vi "CalibrateMultiFlows.vi"(6 "Base Dilution":dbl=0.1, 7 "MFCS_EZ":T4=refnum, 8 "Manual Default Set Pressures":dbl[](array[numeric])=[268.25189208984375, 1037.0302734375, 980.2239990234375, 978.9616088867188], 9 "Missaleneouns Parems":T2={"Ctr Odor Valve"=14, "Water Mix Valve"=12, "Total Odor Flow"=425.0, "Total Flow Setpoint"=531.25, "Control Pressure Channel"=1, "Mix Water Pressure Channel"=2}, 10 "Calibration Refs":T3={"Pressure Controller List"=[2, 2, 2, 3, 4], "Ratio List"=[0.9, 0.7, 0.6, 0.1, 0.1], "Valve List"=[12, 12, 12, 0, 8]}, 11 "Calibration Mode":T5(ring)) -> (0 "Aborted?":bool, 2 "New Manual Pressure":dbl[](array[numeric]), 3 "Set Pressure Cluster":T1)   [LabVIEW 2016]
uses:
  <userlib>/Fluigent/Fluigent MFCS/FluigentMFCS_Full.llb/_EZmfcsRefNum.ctl
  <userlib>/Fluigent/Fluigent MFCS/FluigentMFCS_Full.llb/_EZmfcsEnum.ctl
  <userlib>/Fluigent/Fluigent MFCS/FluigentMFCS_Full.llb/MFCS_EZ Write Channel Pressure.vi
panel:
  out "Set Water Mix Pressures":dbl[](array[numeric])
  out "Control Pressure":dbl=268.25189208984375
  out "odor Starting Pressure":dbl=980.2239990234375
  out "Water Mix Starting PRessure":dbl=1037.0302734375
  out "Ctr Starting Pressure":dbl=268.25189208984375
  out "Set Odor Pressures":dbl[](array[numeric])
  # "Indexed by pressure controller"
  # "indexed by possible ratios"
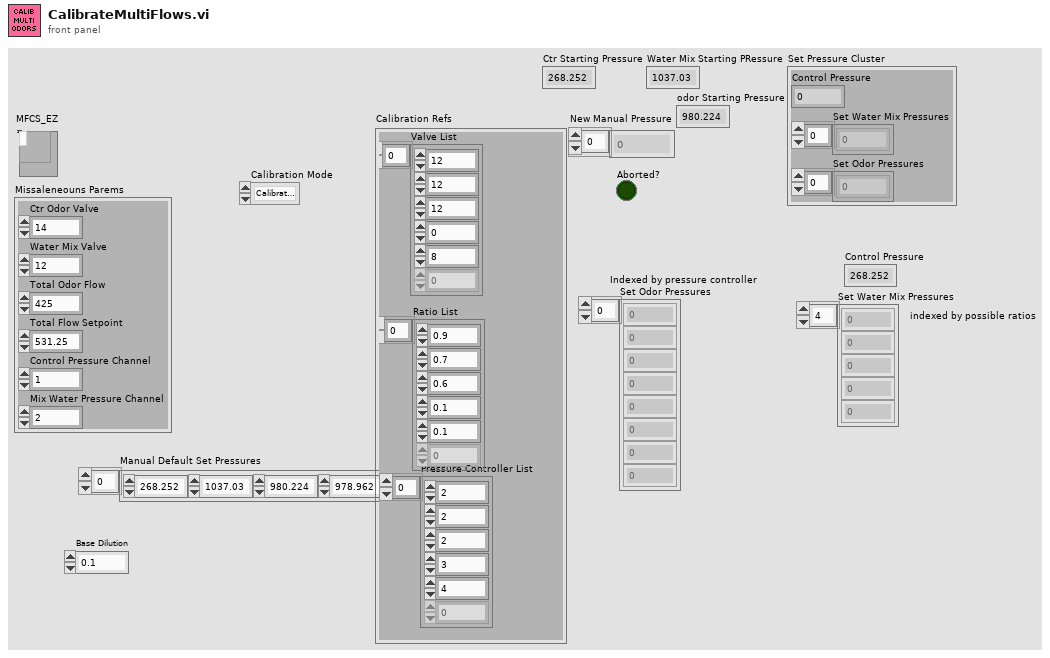
[diagram p1: front panel]
types:
  T1 = cluster{"Control Pressure":dbl, "Set Water Mix Pressures":dbl[], "Set Odor Pressures":dbl[]}
  T2 = cluster{"Ctr Odor Valve":u16, "Water Mix Valve":u16, "Total Odor Flow":dbl, "Total Flow Setpoint":dbl, "Control Pressure Channel":u16, "Mix Water Pressure Channel":u16}
  T3 = cluster{"Pressure Controller List":u8[], "Ratio List":dbl[], "Valve List":u16[]}
  T4 = typedef "_EZmfcsRefNum.ctl" = refnum<k1>
  T5 = enum16{"Calibrate All", "Control Only", "Odors Only"}
  T6 = cluster{"Ratio":dbl, "Valve":u16, "Pressure Channel":u8}[]
  T7 = cluster{"Flowboards":enum16{"A", "B", "C"}[], "Channels":enum16{"1", "2", "3", "4", "5", "6", "7", "8"}[], "States":bool[]}
  T8 = enum16{"Release", "Create", "Send", "Wait", "Cancel"}
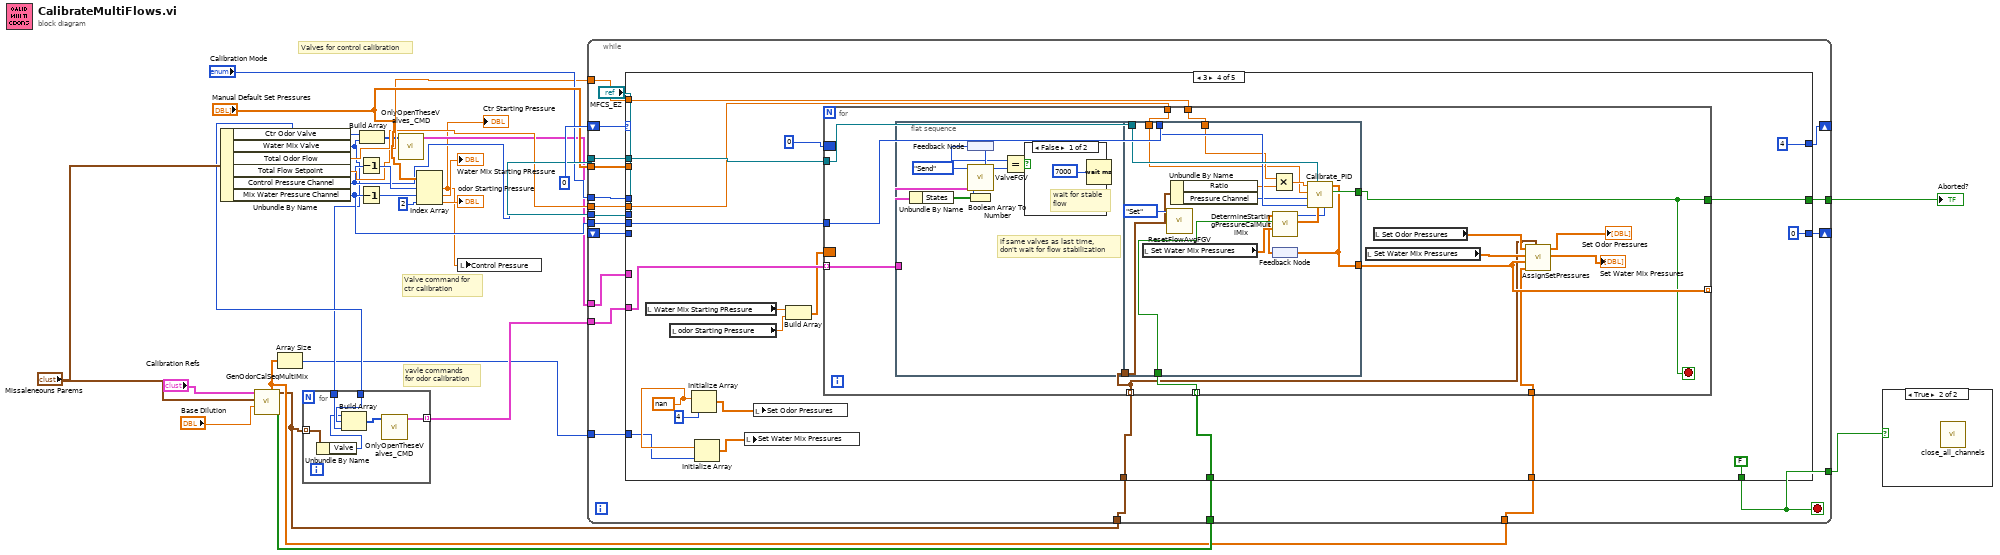
[diagram p0: block diagram]
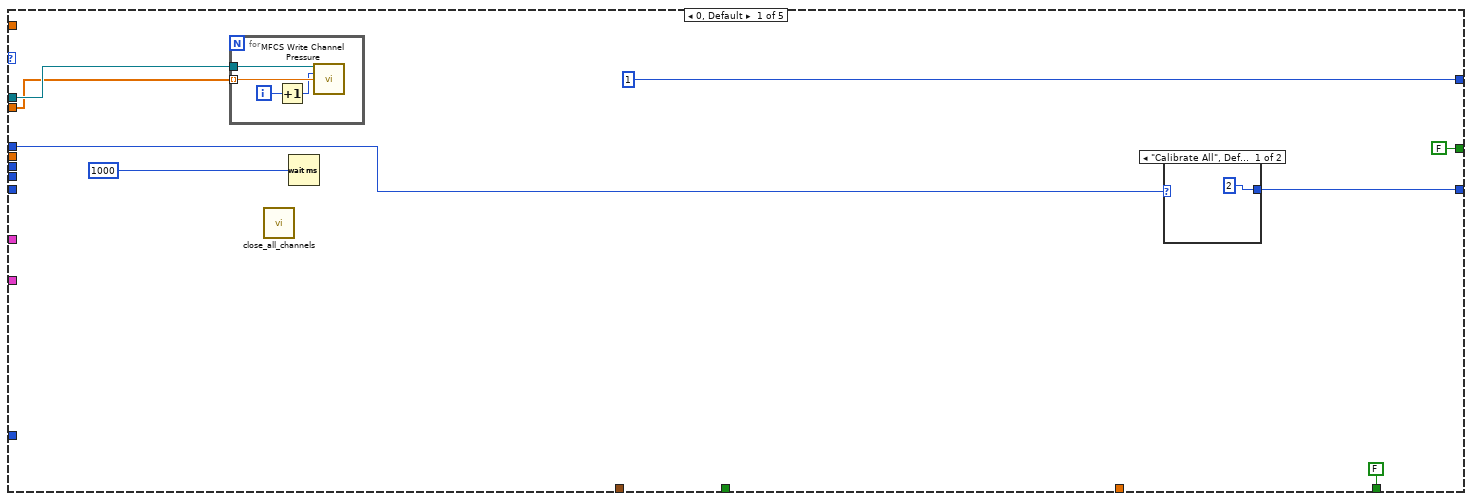
[diagram p3: hidden frame]
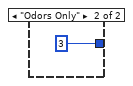
[diagram p4: hidden frame]
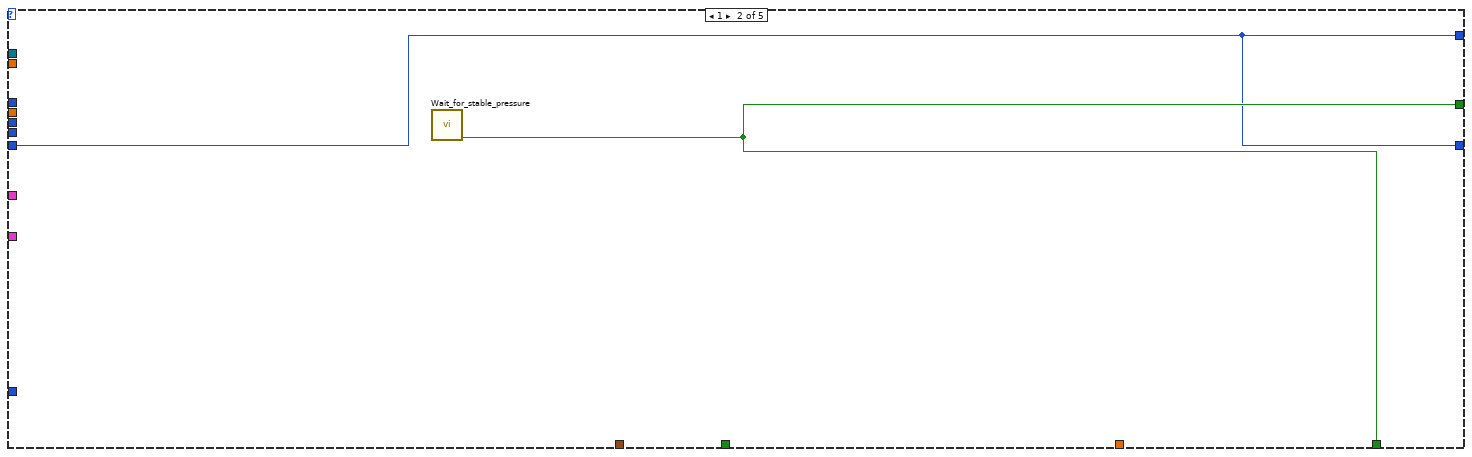
[diagram p5: hidden frame]
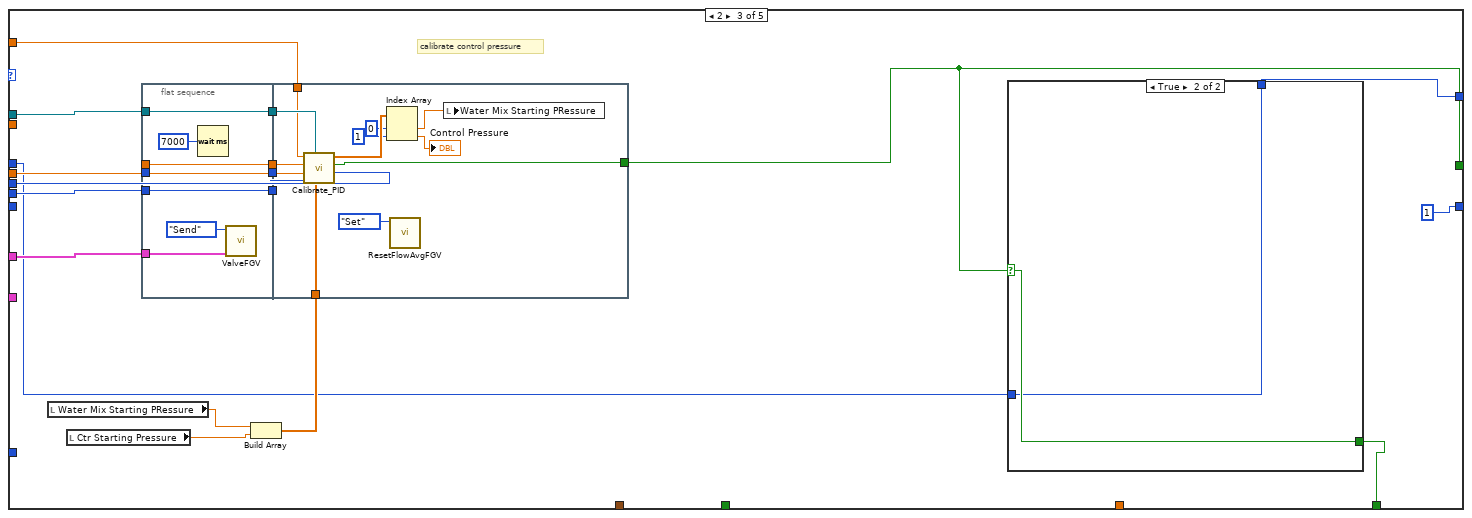
[diagram p6: hidden frame]
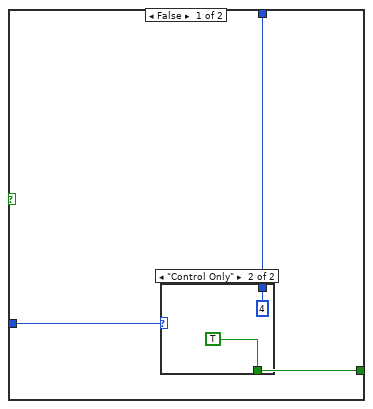
[diagram p7: hidden frame]
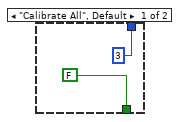
[diagram p8: hidden frame]
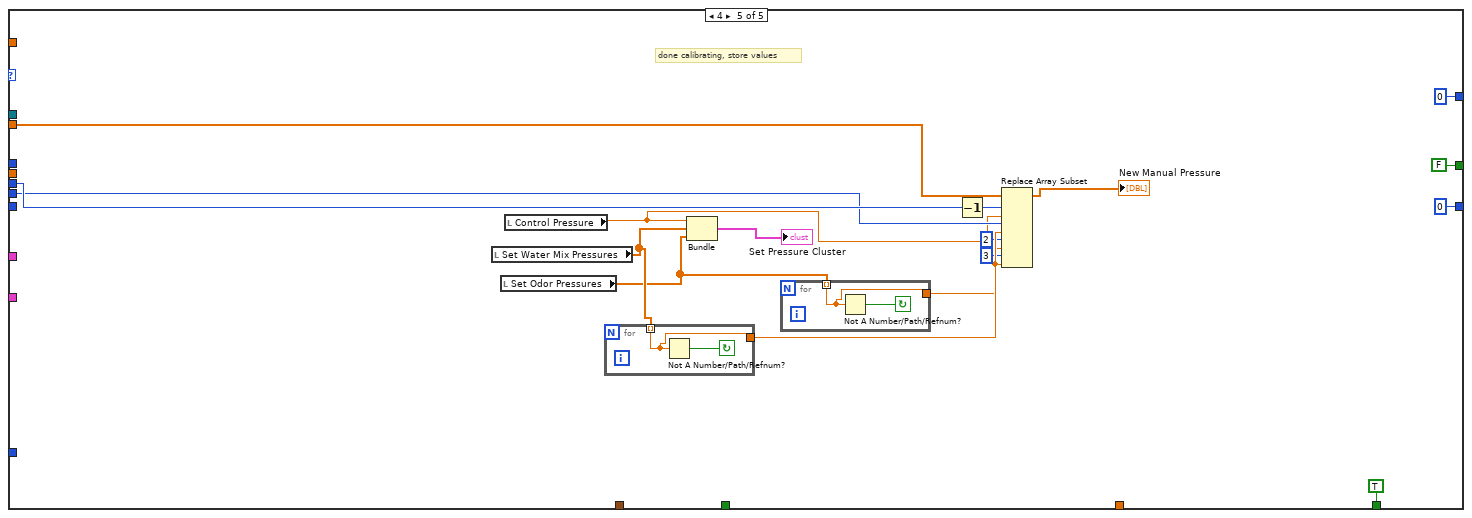
[diagram p10: hidden frame]
diagram:
  # "vavle commands\nfor odor calibration"
  # "Valve command for \nctr calibration"
  # "Valves for control calibration"
  n1 = Unbundle By Name("Missaleneouns Parems") -> ("Ctr Odor Valve"=w8:u16, "Water Mix Valve"=w7:u16, "Total Odor Flow"=w18:dbl, "Total Flow Setpoint"=w17:dbl, "Control Pressure Channel"=w16:u16, "Mix Water Pressure Channel"=w15:u16)
  n2 = call "GenOdorCalSeqMultiMix.vi"("Base Dilution"="Base Dilution", "Missaleneouns Parems"="Missaleneouns Parems", "Calibration Refs"="Calibration Refs") -> ("newRatio"=w5:bool[], "Cal Ref OUt"=w2:T6, "Possible Water Mix Ratios"=w4:dbl[])  [unwired: 5 in, 1 out]
  n3 = Array Size(array=w4) -> (size(s)=w3:i32)
  n4 = for {
    tunnel: w8 -> [w34]
    tunnel: w7 -> [w33]
    tunnel: [w31] -> w6 mode=indexing
    tunnel: w2 -> [w30] mode=indexing
    n5 = Unbundle By Name(w30) -> ("Valve"=w29:u16)
    n6 = Build Array(w29, w34, w33) -> (w32:u16[])
    n7 = call "OnlyOpenTheseValves_CMD.vi"("Valve List"=w32) -> ("Valve Comand"=w31:T7)  [unwired: 10 in]
  }
  n8 = Decrement(x=w16) -> (x-1=w24:u16)
  n9 = Decrement(x=w15) -> (x-1=w25:u16)
  n10 = Build Array(w8, w7) -> (w14:u16[])
  n11 = call "OnlyOpenTheseValves_CMD.vi"("Valve List"=w14) -> ("Valve Comand"=w13:T7)  [unwired: 10 in]
  n12 = Index Array(array="Manual Default Set Pressures", index #1=w24, index #2=w25, index #3=2 ("index")) -> (element #1=w1:dbl, element #2=→"Water Mix Starting PRessure":dbl, element #3=→"odor Starting Pressure":dbl)
  "Ctr Starting Pressure" <- w1
  n13 = local write "Control Pressure"(w1) -> ()
  n14 = while {
    shift-right: [w50] -> _
    shift-left: 0 -> [w53]
    tunnel: "MFCS_EZ" -> [w52]
    tunnel: "Manual Default Set Pressures" -> [w51]
    tunnel: "Calibration Mode" -> [w49]
    shift-right: [w48] -> _
    shift-left: _ -> [w46]
    tunnel: [w47] -> w19
    tunnel: w18 -> [w45]
    tunnel: w17 -> [w44]
    tunnel: w16 -> [w35]
    tunnel: w15 -> [w43]
    tunnel: w13 -> [w42]
    tunnel: [w41] -> w12
    tunnel: w6 -> [w40]
    tunnel: w2 -> [w39]
    tunnel: w5 -> [w38]
    tunnel: w4 -> [w37]
    tunnel: w3 -> [w36]
    stop <- w41 stop-if-true
    n15 = case shown="3" w53 {
      tunnel: w52 -> [w61 _ w87 w135 _]
      tunnel: w51 -> [w60 _ _ _ w184]
      tunnel: [1 w68 w71 4 0] -> w50
      tunnel: w49 -> [w57 _ w74 _ _]
      tunnel: [w56 w68 1 0 0] -> w48
      tunnel: [FALSE ("Aborted?") w69 w70 w119 FALSE ("Aborted?")] -> w47
      tunnel: [FALSE ("Aborted?") w69 w73 FALSE ("Aborted?") TRUE ("Aborted?")] -> w41
      tunnel: w46 -> [_ w68 _ _ _]
      tunnel: w45 -> [_ _ w86 w134 _]
      tunnel: w44 -> [_ _ w85 w133 _]
      tunnel: w35 -> [_ _ w84 _ w183]
      tunnel: w43 -> [_ _ w83 w131 w181]
      tunnel: w42 -> [_ _ w75 _ _]
      tunnel: w40 -> [_ _ _ w137 _]
      tunnel: w39 -> [_ _ _ w132 _]
      tunnel: w38 -> [_ _ _ w127 _]
      tunnel: w37 -> [_ _ _ w126 _]
      tunnel: w36 -> [_ _ _ w121 _]
      frame 0, Default {
        n16 = for {
          tunnel: w60 -> [w67] mode=indexing
          tunnel: w61 -> [w65]
          i -> [w66]
          n17 = Increment(x=w66) -> (x+1=w64:i32)
          n18 = call-poly <userlib>:"MFCS Write Channel Pressure.vi"("MFCS_EZ"=w65, "Channel Number (default=1)"=w64, "Pressure (mBar)"=w67) -> ()  [unwired: 11 in, 2 out]
        }
        n19 = call "close_all_channels.vi"() -> ()  [unwired: 12 in]
        n20 = Wait (ms)(milliseconds to wait=u32 1000) -> ()  [unwired: 1 out]
        n21 = case shown="\"Calibrate All\", Default" w57 {
          tunnel: [2 3] -> w56
          frame "Calibrate All", Default {
          }
          frame "Odors Only" {
          }
        }
      }
      frame 1 {
        n22 = call "Wait_for_stable_pressure.vi"() -> ("Aborted?"=w69:bool)  [unwired: 8 in, 1 out]
      }
      frame 2 {
        # "calibrate control pressure"
        n23 = local read "Water Mix Starting PRessure"() -> (w82:dbl)
        n24 = local read "Ctr Starting Pressure"() -> (w81:dbl)
        n25 = flat-sequence {
          tunnel: w83 -> [w100]
          tunnel: w84 -> [w101]
          tunnel: w85 -> [w102]
          tunnel: w87 -> [w103]
          tunnel: [w103] -> w79
          tunnel: [w102] -> w78
          tunnel: [w101] -> w77
          tunnel: [w100] -> w76
          tunnel: w75 -> [w98]
          tunnel: [w115] -> w70
          tunnel: w86 -> [w114]
          tunnel: w80 -> [w110]
          tunnel: w79 -> [w116]
          tunnel: w78 -> [w113]
          tunnel: w77 -> [w112]
          tunnel: w76 -> [w111]
          frame #0 {
            n26 = Wait (ms)(milliseconds to wait=u32 7000) -> ()  [unwired: 1 out]
            n27 = call "ValveFGV.vi"("Valve Data"=w98, "Action"=T8."Send") -> ()  [unwired: 6 in, 4 out]
          }
          frame #1 {
            n28 = call "Calibrate_PID.vi"("Starting Pressure"=w110, "MFCS_EZ"=w116, "Water Mix Pressure Channel"=w111, "Odor Mix Pressure Channel"=w112, "Ftot Setpoint"=w113, "F1 Setpoint"=w114) -> ("Aborted?"=w115:bool, "Set Pressure Out"=w108:dbl[])  [unwired: 4 in]
            n29 = Index Array(array=w108, index #1=0 ("index"), index #2=1 ("index")) -> (element #1=w104:dbl, element #2=→"Control Pressure":dbl)
            n30 = call "ResetFlowAvgFGV.vi"("Action"=enum16{"Create", "Set", "Wait"}."Set") -> ()  [unwired: 10 in, 1 out]
            n31 = local write "Water Mix Starting PRessure"(w104) -> ()
          }
        }
        n32 = Build Array(w82, w81) -> (w80:dbl[])
        n33 = case shown="True" w70 {
          selector: w70 -> [_ w96]
          tunnel: w74 -> [w90 w95]
          tunnel: [w89 w96] -> w73
          tunnel: [w88 w95] -> w71
          frame False {
            n34 = case shown="\"Control Only\"" w90 {
              tunnel: [FALSE TRUE] -> w89
              tunnel: [3 4] -> w88
              frame "Calibrate All", Default {
              }
              frame "Control Only" {
              }
            }
          }
          frame True {
          }
        }
      }
      frame 3 {
        w122 = nan
        n35 = local read "Water Mix Starting PRessure"() -> (w130:dbl)
        n36 = local read "odor Starting Pressure"() -> (w128:dbl)
        n37 = Initialize Array(w122, 4 ("dimension size")) -> (w124:dbl[])
        n38 = Initialize Array(w122, w121) -> (w125:dbl[])
        n39 = local write "Set Water Mix Pressures"(w125) -> ()
        n40 = local write "Set Odor Pressures"(w124) -> ()
        n41 = Build Array(w130, w128) -> (w129:dbl[])
        n42 = for {
          tunnel: w137 -> [w151] mode=indexing
          border: u32 0 -> [_]
          tunnel: w135 -> [w150]
          tunnel: w134 -> [w149]
          tunnel: w133 -> [w148]
          tunnel: w132 -> [w141] mode=indexing
          tunnel: w131 -> [w147]
          tunnel: [w143] -> _ mode=indexing
          border: w129 -> [_]
          tunnel: w127 -> [w146] mode=indexing
          tunnel: w126 -> [w142]
          tunnel: [w138] -> w119
          stop <- w138 stop-if-true
          n43 = flat-sequence {
            tunnel: w151 -> [w156]
            tunnel: [w174] -> w138
            tunnel: w150 -> [w172]
            tunnel: w149 -> [w160]
            tunnel: w148 -> [w159]
            tunnel: w141 -> [w164]
            tunnel: w147 -> [w171]
            tunnel: [w170] -> w143
            tunnel: w146 -> [w169]
            frame #0 {
              # "if same valves as last time, \ndon't wait for flow stabilization"
              n44 = Unbundle By Name(w156) -> ("States"=w155:bool[])
              n45 = feedback #1() -> (w153:u32)
              n46 = call "ValveFGV.vi"("Valve Data"=w156, "Action"=T8."Send") -> ()  [unwired: 6 in, 4 out]
              n47 = Boolean Array To Number(Boolean array=w155) -> (number=w154:u32)
              n48 = feedback-in #1(w154) -> ()
              n49 = Equal?(x=w153, y=w154) -> (x = y?=w152:bool)
              n50 = case shown="False" w152 {
                frame False {
                  # "wait for stable\nflow"
                  n51 = Wait (ms)(milliseconds to wait=u32 7000) -> ()  [unwired: 1 out]
                }
                frame True {
                }
              }
            }
            frame #1 {
              n52 = local read "Set Water Mix Pressures"() -> (w168:dbl[])
              n53 = call "ResetFlowAvgFGV.vi"("Action"=enum16{"Create", "Set", "Wait"}."Set") -> ()  [unwired: 10 in, 1 out]
              n54 = Unbundle By Name(w164) -> ("Ratio"=w163:dbl, "Pressure Channel"=w161:u8)
              n55 = Multiply(x=w160, y=w163) -> (x*y=w162:dbl)
              n56 = feedback #2() -> (w167:dbl[])
              n57 = call "DetermineStartingPressureCalMultiMix.vi"("Set Water Mix Pressures"=w168, "New Ratio?"=w169, "Previous Starting Pressure"=w167) -> ("Starting Pressure"=w166:dbl[], "Which Channel To Control"=w165:enum16{"Odor Chan", "Water Chan", "Both"})  [unwired: 7 in]
              n58 = call "Calibrate_PID.vi"("Which Channel To Control"=w165, "Starting Pressure"=w166, "MFCS_EZ"=w172, "Water Mix Pressure Channel"=w171, "Odor Mix Pressure Channel"=w161, "Ftot Setpoint"=w159, "F1 Setpoint"=w162) -> ("Aborted?"=w174:bool, "Set Pressure Out"=w170:dbl[])  [unwired: 3 in]
              n59 = feedback-in #2(w170) -> ()
            }
          }
          n60 = local read "Set Water Mix Pressures"() -> (w145:dbl[])
          n61 = local read "Set Odor Pressures"() -> (w144:dbl[])
          n62 = call "AssignSetPressures.vi"("Cal Ref"=w141, "Possible Water Mix Ratios"=w142, "New Set Pressures"=w143, "Set Water Mix Pressures In"=w145, "Set Odor Pressures In"=w144) -> ("Set Water Mix Pressures"=→"Set Water Mix Pressures":dbl[], "Set Odor Pressures"=→"Set Odor Pressures":dbl[])  [unwired: 5 in]
        }
      }
      frame 4 {
        # "done calibrating, store values"
        n63 = local read "Set Water Mix Pressures"() -> (w186:dbl[])
        n64 = local read "Set Odor Pressures"() -> (w185:dbl[])
        n65 = local read "Control Pressure"() -> (w180:dbl)
        n66 = for {
          tunnel: w186 -> [w194] mode=indexing
          tunnel: [w194] -> w179
          stop <- w195 continue-if-true
          n67 = Not A Number/Path/Refnum?(number/path/refnum=w194) -> (NaN/Path/Refnum?=w195:bool)
        }
        n68 = Bundle("Control Pressure"=w180, "Set Water Mix Pressures"=w186, "Set Odor Pressures"=w185) -> (→"Set Pressure Cluster":T1)  [unwired: 1 in]
        n69 = for {
          tunnel: w185 -> [w192] mode=indexing
          tunnel: [w192] -> w176
          stop <- w193 continue-if-true
          n70 = Not A Number/Path/Refnum?(number/path/refnum=w192) -> (NaN/Path/Refnum?=w193:bool)
        }
        n71 = Decrement(x=w183) -> (x-1=w182:u16)
        n72 = Replace Array Subset(array=w184, new element #1=w180, index #1=w182, new element #2=w179, index #2=w181, new element #3=w176, index #3=2 ("index"), new element #4=w176, index #4=3 ("index")) -> (→"New Manual Pressure":dbl[])
      }
    }
  }
  "Aborted?" <- w19
  n73 = case shown="True" w12 {
    frame False {
    }
    frame True {
      n74 = call "close_all_channels.vi"() -> ()  [unwired: 12 in]
    }
  }
